vi "Leak_Comp.vi"(8 "error in":errorcluster, 9 "LeakCompMode":dbl format="%#_13g", 10 "TargetBiasVoltage":dbl format="%_10g", 11 "KeyState":string) -> (0 "error out":errorcluster, 1 "VError":dbl format="%_10g", 2 "ReadCurrent":dbl format="%_10g", 3 "ReadVoltage":dbl format="%_10g", 7 "Voltage Adjusted?":bool)   [LabVIEW 2020]
uses:
  Global 1.vi
panel:
  out "error out : Gate Res":errorcluster
  out "%DiffVoltage":dbl format="%_10g"
  out "Iteration Leak Comp":i32
  in  "MinVError":dbl format="%_10g"
  out "NewBiasVoltage":dbl format="%_10g"
  out "RSeries":dbl format="%#_13g"
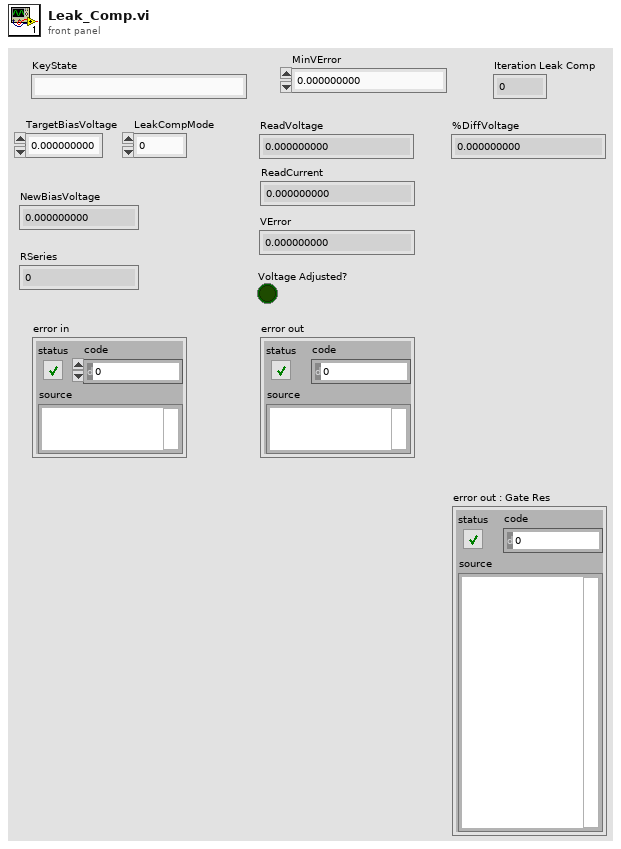
[diagram p1: front panel]
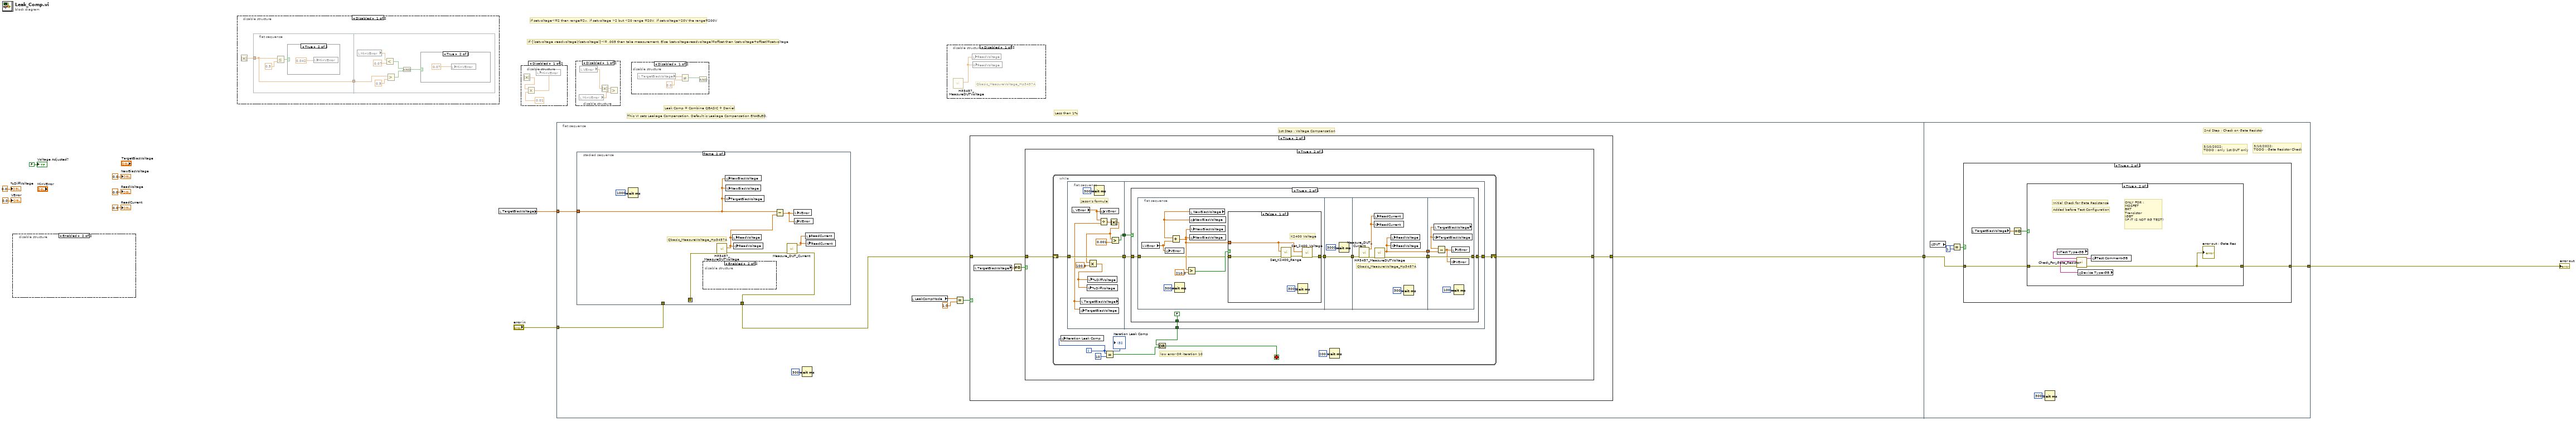
[diagram p0: block diagram]
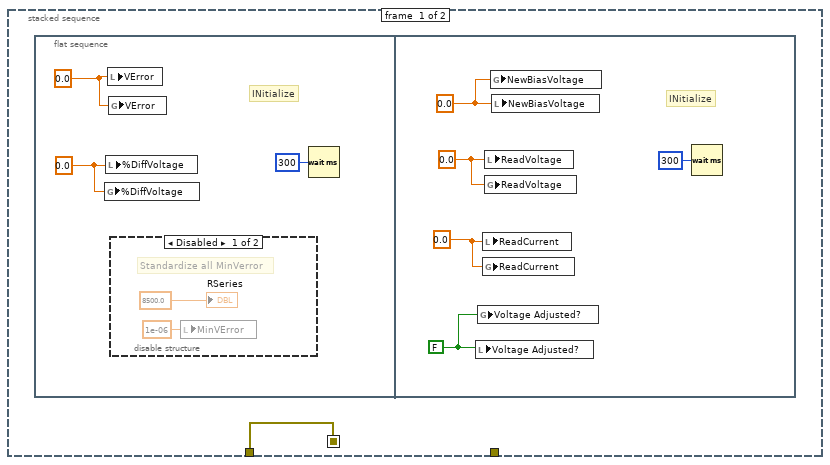
[diagram p2: hidden frame]
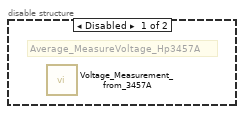
[diagram p4: hidden frame]
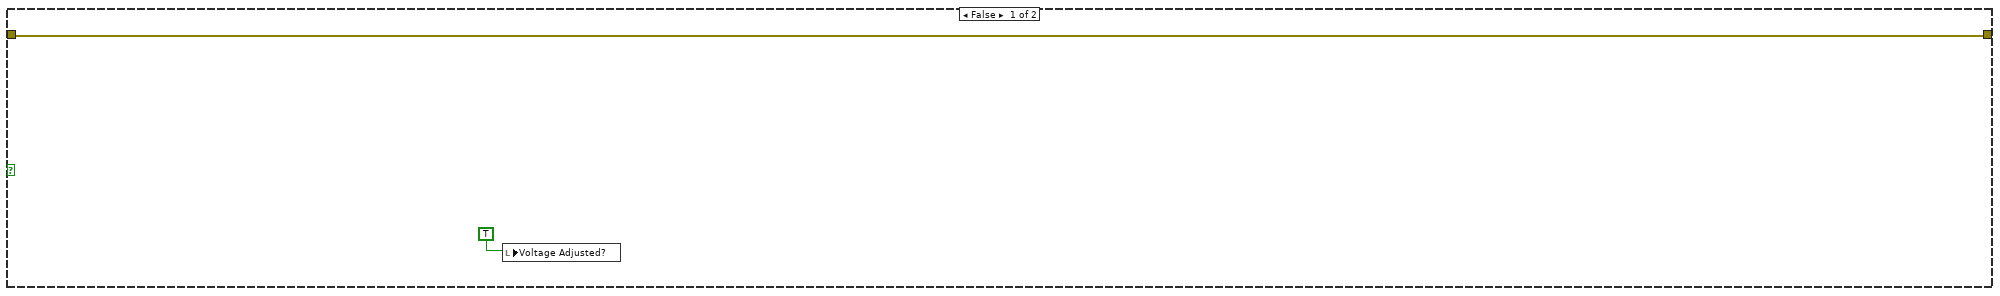
[diagram p5: hidden frame]
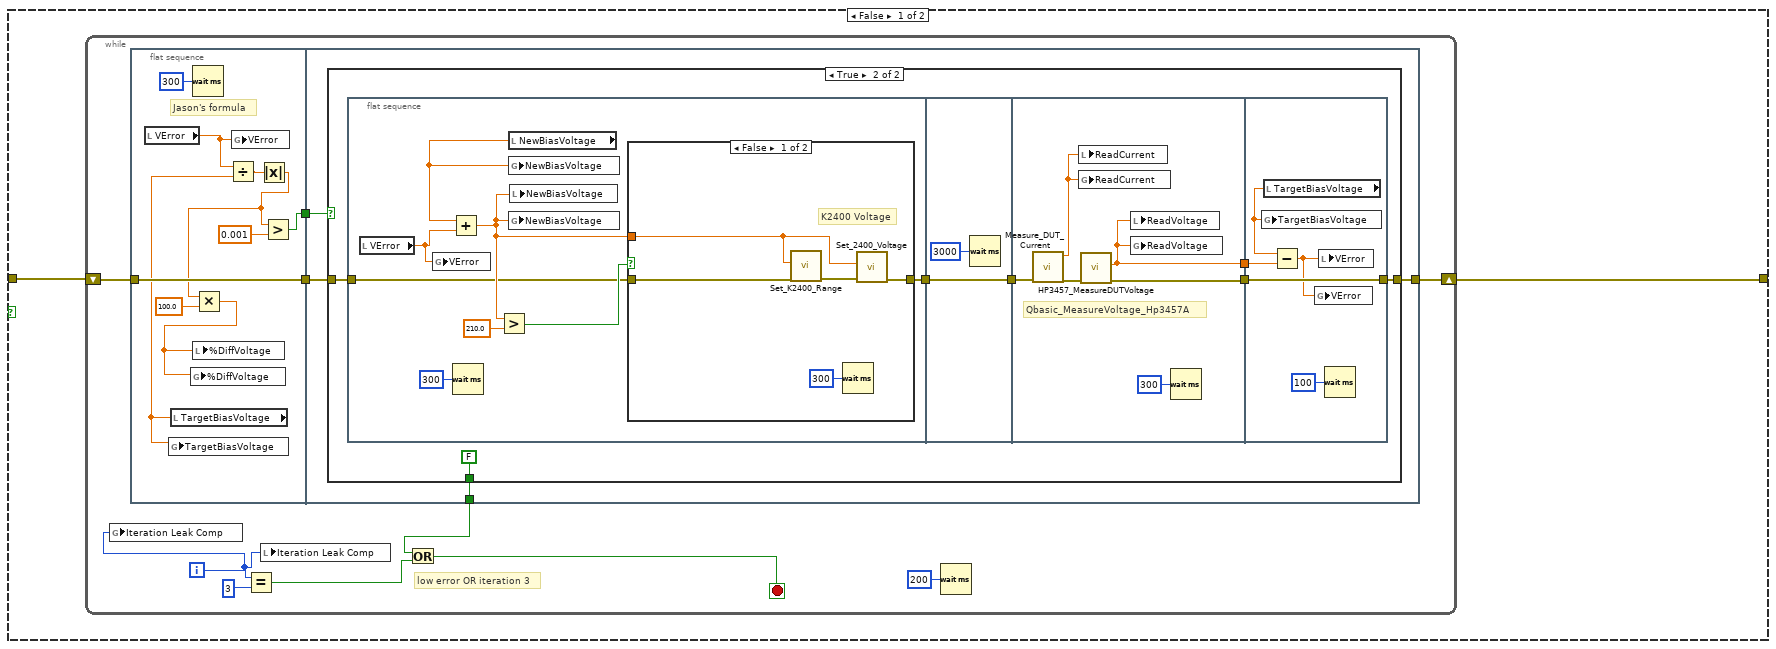
[diagram p6: hidden frame]
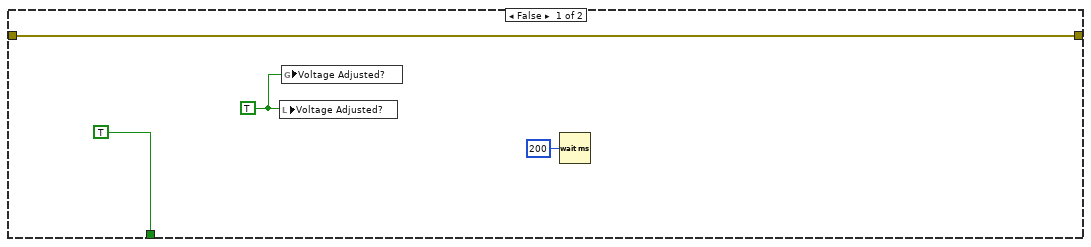
[diagram p7: hidden frame]
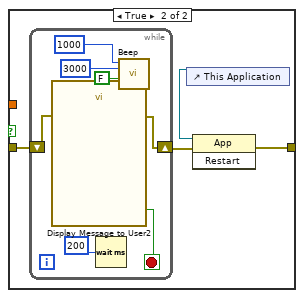
[diagram p8: hidden frame]
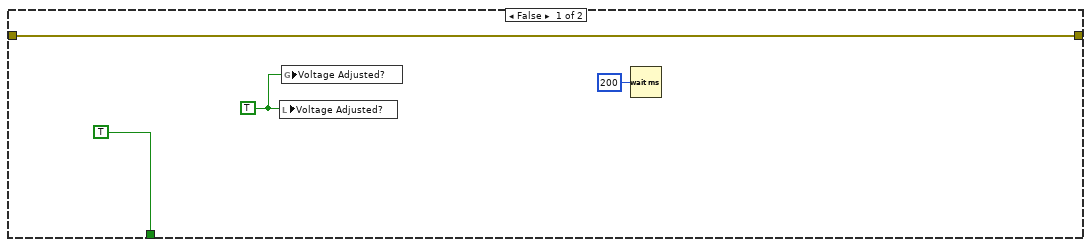
[diagram p9: hidden frame]
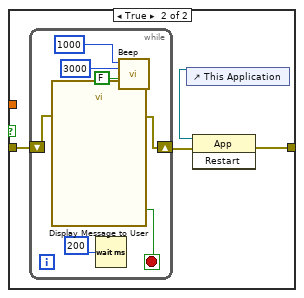
[diagram p10: hidden frame]
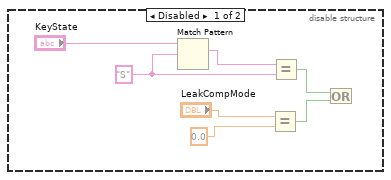
[diagram p20: hidden frame]
diagram:
  # "Less than 1%"
  # "If {(setvoltage -readvoltage)/(setvoltage)}<= .005 then take measurement. Else (setvoltage-readvoltage)=offset then (setvoltage+offset)=setvoltage"
  # "if setvoltage<=2 then range=2v, if setvoltage >2 but <20 range =20V, if setvoltage>20V the range=200V"
  # "Leak Comp = Combine QBASIC + Daniel"
  # "This VI sets Leakage Compensation. Default is Leakage Compensation ENABLED."
  n1 = disable-structure shown="Enabled" {
    frame Disabled {
      w16 = "S" ("regular expression")
      n2 = Match Pattern(string="KeyState", regular expression=w16) -> (match substring=w17:string)  [unwired: 1 in, 3 out]
      n3 = Equal?(x="LeakCompMode", y=0.0) -> (x = y?=w11:bool)
      n4 = Equal?(x=w17, y=w16) -> (x = y?=w14:bool)
      n5 = Or(x=w14, y=w11) -> (x .or. y?=w15:bool)
    }
    frame Enabled {
    }
  }
  n6 = disable-structure shown="Disabled" {
    frame Disabled {
      n7 = Absolute Value() -> (abs(x)=w19:dbl)  [unwired: 1 in]
      n8 = flat-sequence {
        tunnel: w19 -> [w21]
        tunnel: [w21] -> w20
        tunnel: w20 -> [w25]
        frame #0 {
          n9 = Less Or Equal?(x=w21, y=0.5) -> (x <= y?=w23:bool)
          n10 = case shown="True" w23 {
            frame False {
            }
            frame True {
              n11 = local write "MinVError"(0.042) -> ()
            }
          }
        }
        frame #1 {
          n12 = local read "MinVError"() -> (w31:dbl)
          n13 = Less?(x=w31, y=0.07) -> (x < y?=w30:bool)
          n14 = Greater?(x=w25, y=0.5) -> (0:w29:bool)
          n15 = And(x=w30, y=w29) -> (x .and. y?=w28:bool)
          n16 = case shown="True" w28 {
            frame False {
            }
            frame True {
              n17 = local write "MinVError"(0.07 ("MinVError")) -> ()
            }
          }
        }
      }
    }
    frame Enabled {
    }
  }
  n18 = local read "TargetBiasVoltage"() -> (w8:dbl)
  n19 = disable-structure shown="Disabled" {
    frame Disabled {
      n20 = Absolute Value() -> (abs(x)=w33:dbl)  [unwired: 1 in]
      n21 = Multiply(x=w33, y=0.01) -> (x*y=w35:dbl)
      n22 = local write "MinVError"(w35) -> ()
    }
    frame Enabled {
    }
  }
  n23 = flat-sequence {
    tunnel: "error in" -> [w43]
    tunnel: w8 -> [w41]
    tunnel: [w42] -> w7
    tunnel: [w220] -> w9
    tunnel: w7 -> [w221]
    frame #0 {
      # "1st Step : Voltage Compensation"
      n24 = stacked-sequence {
        seq-local: [w44 _] -> [_ w60]
        tunnel: w41 -> [_ w56]
        tunnel: [_ w62] -> w40
        tunnel: w43 -> [w44 _]
        frame #0 {
          n25 = flat-sequence {
            frame #0 {
              w46 = 0.0 ("%DiffVoltage")
              w47 = 0.0
              # "INitialize"
              n26 = global write "Global 1.vi" "%DiffVoltage"(w46) -> ()
              n27 = local write "%DiffVoltage"(w46) -> ()
              n28 = local write "VError"(w47) -> ()
              n29 = global write "Global 1.vi" "VError"(w47) -> ()
              n30 = disable-structure shown="Disabled" {
                frame Disabled {
                  # "Standardize all MinVerror"
                  n31 = local write "MinVError"(1e-06 ("MinVError")) -> ()
                  "RSeries" <- 8500.0
                }
                frame Enabled {
                }
              }
              n32 = Wait (ms)(milliseconds to wait=u32 300) -> ()  [unwired: 1 out]
            }
            frame #1 {
              w51 = FALSE ("Voltage Adjusted?")
              w52 = 0.0 ("ReadVoltage")
              w53 = 0.0 ("ReadCurrent")
              w54 = 0.0 ("NewBiasVoltage")
              # "INitialize"
              n33 = local write "Voltage Adjusted?"(w51) -> ()
              n34 = global write "Global 1.vi" "Voltage Adjusted?"(w51) -> ()
              n35 = local write "ReadCurrent"(w53) -> ()
              n36 = global write "Global 1.vi" "ReadCurrent"(w53) -> ()
              n37 = local write "ReadVoltage"(w52) -> ()
              n38 = global write "Global 1.vi" "ReadVoltage"(w52) -> ()
              n39 = global write "Global 1.vi" "NewBiasVoltage"(w54) -> ()
              n40 = local write "NewBiasVoltage"(w54) -> ()
              n41 = Wait (ms)(milliseconds to wait=u32 300) -> ()  [unwired: 1 out]
            }
          }
        }
        frame #1 {
          # "Qbasic_MeasureVoltage_Hp3457A"
          n42 = Wait (ms)(milliseconds to wait=u32 1000) -> ()  [unwired: 1 out]
          n43 = disable-structure shown="Enabled" {
            frame Disabled {
              # "Average_MeasureVoltage_Hp3457A"
              n44 = call "Voltage_Measurement_from_3457A.vi"() -> ()  [unwired: 10 in, 2 out]
            }
            frame Enabled {
            }
          }
          n45 = call "HP3457_MeasureDUTVoltage.vi"("error in"=w60) -> ("error out"=w61:errorcluster, "DUTVoltage"=w59:dbl)  [unwired: 8 in]
          n46 = global write "Global 1.vi" "NewBiasVoltage"(w56) -> ()
          n47 = global write "Global 1.vi" "TargetBiasVoltage"(w56) -> ()
          n48 = local write "NewBiasVoltage"(w56) -> ()
          n49 = local write "ReadVoltage"(w59) -> ()
          n50 = global write "Global 1.vi" "ReadVoltage"(w59) -> ()
          n51 = Subtract(x=w56, y=w59) -> (x-y=w58:dbl)
          n52 = call "Measure_DUT_Current.vi"("error in"=w61) -> ("error out"=w62:errorcluster, "DUTCurrent"=w57:dbl)  [unwired: 9 in]
          n53 = local write "VError"(w58) -> ()
          n54 = global write "Global 1.vi" "VError"(w58) -> ()
          n55 = local write "ReadCurrent"(w57) -> ()
          n56 = global write "Global 1.vi" "ReadCurrent"(w57) -> ()
        }
      }
      n57 = Wait (ms)(milliseconds to wait=u32 300) -> ()  [unwired: 1 out]
      n58 = local read "LeakCompMode"() -> (w39:dbl)
      n59 = Equal?(x=w39, y=1.0) -> (x = y?=w37:bool)
      n60 = case shown="True" w37 {
        tunnel: w40 -> [w64 w68]
        tunnel: [w64 w67] -> w42
        frame False {
          n61 = local write "Voltage Adjusted?"(TRUE ("Voltage Adjusted?")) -> ()
        }
        frame True {
          n62 = local read "TargetBiasVoltage"() -> (w65:dbl)
          n63 = Not Equal To 0?(x=w65) -> (x != 0?=w66:bool)
          n64 = case shown="True" w66 {
            tunnel: w68 -> [w69 w144]
            tunnel: [w70 w143] -> w67
            frame False {
              n65 = while {
                shift-right: [w79] -> w70
                shift-left: w69 -> [w80]
                i -> [w71]
                stop <- w78 stop-if-true
                # "low error OR iteration 3"
                n66 = global write "Global 1.vi" "Iteration Leak Comp"(w71) -> ()
                n67 = flat-sequence {
                  tunnel: w80 -> [w90]
                  tunnel: [w90] -> w73
                  tunnel: [w88] -> w72
                  tunnel: [w93] -> w79
                  tunnel: [w91] -> w74
                  tunnel: w73 -> [w94]
                  tunnel: w72 -> [w92]
                  frame #0 {
                    # "Jason's formula"
                    n68 = local read "VError"() -> (w87:dbl)
                    n69 = local read "TargetBiasVoltage"() -> (w86:dbl)
                    n70 = global write "Global 1.vi" "TargetBiasVoltage"(w86) -> ()
                    n71 = Wait (ms)(milliseconds to wait=u32 300) -> ()  [unwired: 1 out]
                    n72 = Divide(x=w87, y=w86) -> (x/y=w83:dbl)
                    n73 = global write "Global 1.vi" "VError"(w87) -> ()
                    n74 = Absolute Value(x=w83) -> (abs(x)=w82:dbl)
                    n75 = Multiply(x=w82, y=100.0) -> (x*y=w84:dbl)
                    n76 = global write "Global 1.vi" "%DiffVoltage"(w84) -> ()
                    n77 = local write "%DiffVoltage"(w84) -> ()
                    n78 = Greater?(x=w82, y=0.001) -> (0:w88:bool)
                  }
                  frame #1 {
                    n79 = case shown="True" w92 {
                      tunnel: w94 -> [w98 w104]
                      tunnel: [w98 w103] -> w93
                      tunnel: [TRUE FALSE] -> w91
                      frame False {
                        w96 = TRUE ("Voltage Adjusted?")
                        n80 = local write "Voltage Adjusted?"(w96) -> ()
                        n81 = global write "Global 1.vi" "Voltage Adjusted?"(w96) -> ()
                        n82 = Wait (ms)(milliseconds to wait=u32 200) -> ()  [unwired: 1 out]
                      }
                      frame True {
                        n83 = flat-sequence {
                          tunnel: w104 -> [w108]
                          tunnel: [w113] -> w100
                          tunnel: w100 -> [w131]
                          tunnel: [w131] -> w99
                          tunnel: w99 -> [w137]
                          tunnel: [w135] -> w102
                          tunnel: [w133] -> w101
                          tunnel: [w142] -> w103
                          tunnel: w102 -> [w142]
                          tunnel: w101 -> [w141]
                          frame #0 {
                            n84 = local read "VError"() -> (w110:dbl)
                            n85 = global write "Global 1.vi" "VError"(w110) -> ()
                            n86 = Wait (ms)(milliseconds to wait=u32 300) -> ()  [unwired: 1 out]
                            n87 = local read "NewBiasVoltage"() -> (w107:dbl)
                            n88 = Add(x=w107, y=w110) -> (x+y=w109:dbl)
                            n89 = Greater?(x=w109, y=210.0) -> (0:w111:bool)
                            n90 = global write "Global 1.vi" "NewBiasVoltage"(w107) -> ()
                            n91 = global write "Global 1.vi" "NewBiasVoltage"(w109) -> ()
                            n92 = local write "NewBiasVoltage"(w109) -> ()
                            n93 = case shown="False" w111 {
                              tunnel: [w118 w119] -> w113
                              tunnel: w109 -> [w115 _]
                              tunnel: w108 -> [w117 w122]
                              frame False {
                                # "K2400 Voltage"
                                n94 = call "Set_K2400_Range.vi"("error in (no error)"=w117, "Desired Voltage"=w115) -> ("error out"=w116:errorcluster)  [unwired: 9 in]
                                n95 = Wait (ms)(milliseconds to wait=u32 300) -> ()  [unwired: 1 out]
                                n96 = call "Set_2400_Voltage.vi"("error in"=w116, "Voltage"=w115) -> ("error out"=w118:errorcluster)  [unwired: 8 in]
                              }
                              frame True {
                                n97 = while {
                                shift-right: [w127] -> w120
                                shift-left: w122 -> [w129]
                                stop <- w128 stop-if-true
                                n98 = call "Display Message to User2"("error in (no error)"=w129) -> ("error out"=w127:errorcluster, "OK"=w128:bool)  [unwired: 9 in]
                                n99 = Wait (ms)(milliseconds to wait=u32 200) -> ()  [unwired: 1 out]
                                n100 = call <vilib>:"Beep.vi"("use system alert? (T)"=FALSE, "duration (msec)"=u32 3000, "frequency (Hz)"=u32 1000) -> ()  [unwired: 9 in]
                                }
                                n101 = control-ref of="This Application"() -> (w121:refnum<vi>)
                                n102 = invoke class="App" method="Restart"(reference=w121, error in=w120) -> (error out=w119:errorcluster)  [unwired: 1 in, 2 out]
                              }
                            }
                          }
                          frame #1 {
                            n103 = Wait (ms)(milliseconds to wait=u32 3000) -> ()  [unwired: 1 out]
                          }
                          frame #2 {
                            # "Qbasic_MeasureVoltage_Hp3457A"
                            n104 = call "Measure_DUT_Current.vi"("error in"=w137) -> ("error out"=w136:errorcluster, "DUTCurrent"=w134:dbl)  [unwired: 9 in]
                            n105 = local write "ReadCurrent"(w134) -> ()
                            n106 = global write "Global 1.vi" "ReadCurrent"(w134) -> ()
                            n107 = call "HP3457_MeasureDUTVoltage.vi"("error in"=w136) -> ("error out"=w135:errorcluster, "DUTVoltage"=w133:dbl)  [unwired: 8 in]
                            n108 = local write "ReadVoltage"(w133) -> ()
                            n109 = global write "Global 1.vi" "ReadVoltage"(w133) -> ()
                            n110 = Wait (ms)(milliseconds to wait=u32 300) -> ()  [unwired: 1 out]
                          }
                          frame #3 {
                            n111 = local read "TargetBiasVoltage"() -> (w140:dbl)
                            n112 = global write "Global 1.vi" "TargetBiasVoltage"(w140) -> ()
                            n113 = Subtract(x=w140, y=w141) -> (x-y=w139:dbl)
                            n114 = global write "Global 1.vi" "VError"(w139) -> ()
                            n115 = local write "VError"(w139) -> ()
                            n116 = Wait (ms)(milliseconds to wait=u32 100) -> ()  [unwired: 1 out]
                          }
                        }
                      }
                    }
                  }
                }
                n117 = Equal?(x=w71, y=3 ("x")) -> (x = y?=w75:bool)
                n118 = local write "Iteration Leak Comp"(w71) -> ()
                n119 = Or(x=w74, y=w75) -> (x .or. y?=w78:bool)
                n120 = Wait (ms)(milliseconds to wait=u32 200) -> ()  [unwired: 1 out]
              }
            }
            frame True {
              n121 = while {
                shift-right: [w153] -> w143
                shift-left: w144 -> [w154]
                i -> [w145]
                stop <- w152 stop-if-true
                # "low error OR iteration 10"
                n122 = global write "Global 1.vi" "Iteration Leak Comp"(w145) -> ()
                n123 = flat-sequence {
                  tunnel: w154 -> [w164]
                  tunnel: [w164] -> w147
                  tunnel: [w162] -> w146
                  tunnel: [w167] -> w153
                  tunnel: [w165] -> w148
                  tunnel: w147 -> [w168]
                  tunnel: w146 -> [w166]
                  frame #0 {
                    # "Jason's formula"
                    n124 = local read "VError"() -> (w161:dbl)
                    n125 = local read "TargetBiasVoltage"() -> (w160:dbl)
                    n126 = global write "Global 1.vi" "TargetBiasVoltage"(w160) -> ()
                    n127 = Wait (ms)(milliseconds to wait=u32 300) -> ()  [unwired: 1 out]
                    n128 = Divide(x=w161, y=w160) -> (x/y=w157:dbl)
                    n129 = global write "Global 1.vi" "VError"(w161) -> ()
                    n130 = Absolute Value(x=w157) -> (abs(x)=w156:dbl)
                    n131 = Multiply(x=w156, y=100.0) -> (x*y=w158:dbl)
                    n132 = global write "Global 1.vi" "%DiffVoltage"(w158) -> ()
                    n133 = local write "%DiffVoltage"(w158) -> ()
                    n134 = Greater?(x=w156, y=0.001) -> (0:w162:bool)
                  }
                  frame #1 {
                    n135 = case shown="True" w166 {
                      tunnel: w168 -> [w172 w178]
                      tunnel: [w172 w177] -> w167
                      tunnel: [TRUE FALSE] -> w165
                      frame False {
                        w170 = TRUE ("Voltage Adjusted?")
                        n136 = local write "Voltage Adjusted?"(w170) -> ()
                        n137 = global write "Global 1.vi" "Voltage Adjusted?"(w170) -> ()
                        n138 = Wait (ms)(milliseconds to wait=u32 200) -> ()  [unwired: 1 out]
                      }
                      frame True {
                        n139 = flat-sequence {
                          tunnel: w178 -> [w182]
                          tunnel: [w187] -> w174
                          tunnel: w174 -> [w205]
                          tunnel: [w205] -> w173
                          tunnel: w173 -> [w211]
                          tunnel: [w209] -> w176
                          tunnel: [w207] -> w175
                          tunnel: [w216] -> w177
                          tunnel: w176 -> [w216]
                          tunnel: w175 -> [w215]
                          frame #0 {
                            n140 = local read "VError"() -> (w184:dbl)
                            n141 = global write "Global 1.vi" "VError"(w184) -> ()
                            n142 = Wait (ms)(milliseconds to wait=u32 300) -> ()  [unwired: 1 out]
                            n143 = local read "NewBiasVoltage"() -> (w181:dbl)
                            n144 = Add(x=w181, y=w184) -> (x+y=w183:dbl)
                            n145 = Greater?(x=w183, y=210.0) -> (0:w185:bool)
                            n146 = global write "Global 1.vi" "NewBiasVoltage"(w181) -> ()
                            n147 = global write "Global 1.vi" "NewBiasVoltage"(w183) -> ()
                            n148 = local write "NewBiasVoltage"(w183) -> ()
                            n149 = case shown="False" w185 {
                              tunnel: [w192 w193] -> w187
                              tunnel: w183 -> [w189 _]
                              tunnel: w182 -> [w191 w196]
                              frame False {
                                # "K2400 Voltage"
                                n150 = call "Set_K2400_Range.vi"("error in (no error)"=w191, "Desired Voltage"=w189) -> ("error out"=w190:errorcluster)  [unwired: 9 in]
                                n151 = Wait (ms)(milliseconds to wait=u32 300) -> ()  [unwired: 1 out]
                                n152 = call "Set_2400_Voltage.vi"("error in"=w190, "Voltage"=w189) -> ("error out"=w192:errorcluster)  [unwired: 8 in]
                              }
                              frame True {
                                n153 = while {
                                shift-right: [w201] -> w194
                                shift-left: w196 -> [w203]
                                stop <- w202 stop-if-true
                                n154 = call "Display Message to User"("error in (no error)"=w203) -> ("error out"=w201:errorcluster, "OK"=w202:bool)  [unwired: 9 in]
                                n155 = Wait (ms)(milliseconds to wait=u32 200) -> ()  [unwired: 1 out]
                                n156 = call <vilib>:"Beep.vi"("use system alert? (T)"=FALSE, "duration (msec)"=u32 3000, "frequency (Hz)"=u32 1000) -> ()  [unwired: 9 in]
                                }
                                n157 = control-ref of="This Application"() -> (w195:refnum<vi>)
                                n158 = invoke class="App" method="Restart"(reference=w195, error in=w194) -> (error out=w193:errorcluster)  [unwired: 1 in, 2 out]
                              }
                            }
                          }
                          frame #1 {
                            n159 = Wait (ms)(milliseconds to wait=u32 3000) -> ()  [unwired: 1 out]
                          }
                          frame #2 {
                            # "Qbasic_MeasureVoltage_Hp3457A"
                            n160 = call "Measure_DUT_Current.vi"("error in"=w211) -> ("error out"=w210:errorcluster, "DUTCurrent"=w208:dbl)  [unwired: 9 in]
                            n161 = local write "ReadCurrent"(w208) -> ()
                            n162 = global write "Global 1.vi" "ReadCurrent"(w208) -> ()
                            n163 = call "HP3457_MeasureDUTVoltage.vi"("error in"=w210) -> ("error out"=w209:errorcluster, "DUTVoltage"=w207:dbl)  [unwired: 8 in]
                            n164 = local write "ReadVoltage"(w207) -> ()
                            n165 = global write "Global 1.vi" "ReadVoltage"(w207) -> ()
                            n166 = Wait (ms)(milliseconds to wait=u32 300) -> ()  [unwired: 1 out]
                          }
                          frame #3 {
                            n167 = local read "TargetBiasVoltage"() -> (w214:dbl)
                            n168 = global write "Global 1.vi" "TargetBiasVoltage"(w214) -> ()
                            n169 = Subtract(x=w214, y=w215) -> (x-y=w213:dbl)
                            n170 = global write "Global 1.vi" "VError"(w213) -> ()
                            n171 = local write "VError"(w213) -> ()
                            n172 = Wait (ms)(milliseconds to wait=u32 100) -> ()  [unwired: 1 out]
                          }
                        }
                      }
                    }
                  }
                }
                n173 = Equal?(x=w145, y=10 ("x")) -> (x = y?=w149:bool)
                n174 = Or(x=w148, y=w149) -> (x .or. y?=w152:bool)
                n175 = Wait (ms)(milliseconds to wait=u32 200) -> ()  [unwired: 1 out]
                "Iteration Leak Comp" <- w145
              }
            }
          }
        }
      }
    }
    frame #1 {
      # "3/10/2022:\nTODO : only 1st DUT only"
      # "3/10/2022:\nTODO : Gate Resistor Check"
      # "2nd Step : Check on Gate Resistor"
      n176 = global read "Global 1.vi" "DUT"() -> (w218:i32)
      n177 = Equal?(x=w218, y=1) -> (x = y?=w219:bool)
      n178 = case shown="True" w219 {
        tunnel: w221 -> [w223 w227]
        tunnel: [w223 w226] -> w220
        frame False {
        }
        frame True {
          n179 = local read "TargetBiasVoltage"() -> (w224:dbl)
          n180 = Equal To 0?(x=w224) -> (x = 0?=w225:bool)
          n181 = case shown="True" w225 {
            tunnel: w227 -> [w228 w230]
            tunnel: [w228 w229] -> w226
            frame False {
            }
            frame True {
              # "ONLY FOR :\nMOSFET\nBRT\nTransistor\nIGBT\n(IF IT IS NOT RG TEST)"
              # "Initial Check for Gate Resistance"
              # "Added before Test Configuration"
              n182 = global read "Global 1.vi" "Test Type-GB"() -> (w233:string)
              n183 = global read "Global 1.vi" "Device Type-GB"() -> (w231:string)
              n184 = call "Check_For_Gate_Resistor.vi"("error in"=w230, "Device Type"=w231, "FET Test Configuration"=w233) -> ("error out"=w229:errorcluster, "Test Comment"=w232:string)  [unwired: 6 in, 1 out]
              "error out : Gate Res" <- w229
              n185 = global write "Global 1.vi" "Test Comment-GB"(w232) -> ()
            }
          }
        }
      }
      n186 = Wait (ms)(milliseconds to wait=u32 300) -> ()  [unwired: 1 out]
    }
  }
  n187 = disable-structure shown="Disabled" {
    frame Disabled {
      n188 = local read "MinVError"() -> (w234:dbl)
      n189 = local read "VError"() -> (w235:dbl)
      n190 = Absolute Value(x=w235) -> (abs(x)=w236:dbl)
      n191 = Greater?(x=w236, y=w234) -> ()  [unwired: 1 out]
    }
    frame Enabled {
    }
  }
  n192 = disable-structure shown="Disabled" {
    frame Disabled {
      n193 = local read "TargetBiasVoltage"() -> (w239:dbl)
      n194 = Not Equal?(x=w239, y=0.0) -> (x != y?=w238:bool)
      n195 = Compound Arithmetic op=AND(w238) -> ()  [unwired: 1 in, 1 out]
    }
    frame Enabled {
    }
  }
  n196 = disable-structure shown="Disabled" {
    frame Disabled {
      # "Qbasic_MeasureVoltage_Hp3457A"
      n197 = call "HP3457_MeasureDUTVoltage.vi"() -> ("DUTVoltage"=w240:dbl)  [unwired: 9 in, 1 out]
      n198 = local write "ReadVoltage"(w240) -> ()
      n199 = global write "Global 1.vi" "ReadVoltage"(w240) -> ()
    }
    frame Enabled {
    }
  }
  "Voltage Adjusted?" <- FALSE ("Voltage Adjusted?")
  "error out" <- w9
  "NewBiasVoltage" <- 0.0 ("NewBiasVoltage")
  "ReadVoltage" <- 0.0 ("ReadVoltage")
  "ReadCurrent" <- 0.0 ("ReadCurrent")
  "VError" <- 0.0 ("VError")
  "%DiffVoltage" <- 0.0 ("%DiffVoltage")
